vi "VFP Network matchSourceINISettingHandler.vi"(8 "error in (no error)":errorcluster, 10 "write Value":bool=TRUE, 11 "Opperation":enum16{"writeKey", "ReadKey"}(ring)=enum."ReadKey") -> (0 "error IO":errorcluster, 2 "read value":bool)   [LabVIEW 2016]
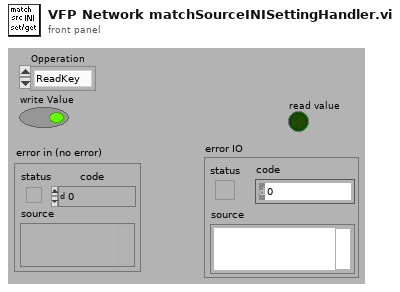
[diagram p1: front panel]
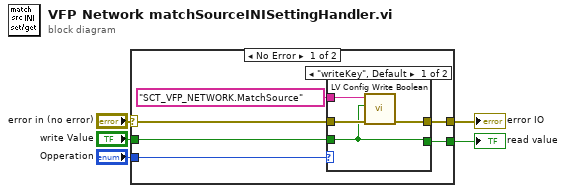
[diagram p0: block diagram]
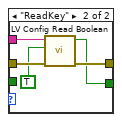
[diagram p2: hidden frame]
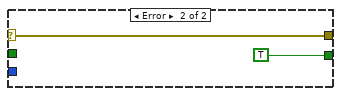
[diagram p3: hidden frame]
diagram:
  n1 = case shown="No Error" "error in (no error)" {
    selector: "error in (no error)" -> [w7 w22]
    tunnel: "Opperation" -> [w11 _]
    tunnel: [w9 TRUE ("value")] -> w5
    tunnel: [w6 w22] -> w4
    tunnel: "write Value" -> [w8 _]
    frame No Error {
      n2 = case shown="\"writeKey\", Default" w11 {
        tunnel: "SCT_VFP_NETWORK.MatchSource" ("key") -> [w13 w17]
        tunnel: w7 -> [w15 w20]
        tunnel: [w12 w16] -> w9
        tunnel: [w14 w19] -> w6
        tunnel: w8 -> [w12 _]
        frame "writeKey", Default {
          n3 = call <resource>:"LV Config Write Boolean.vi"("error in (no error)"=w15, "value"=w12, "key"=w13) -> ("error out"=w14:errorcluster)  [unwired: 4 in]
        }
        frame "ReadKey" {
          n4 = call <resource>:"LV Config Read Boolean.vi"("error in"=w20, "default value"=TRUE, "key"=w17) -> ("error out"=w19:errorcluster, "value"=w16:bool)  [unwired: 2 in, 1 out]
        }
      }
    }
    frame Error {
    }
  }
  "error IO" <- w4
  "read value" <- w5
